vi "WriteFlattenImageOptions.vi"(8 "error in":errorcluster, 9 "Type of Flatten":T1 items=["Image", "Image and Vision Info", "Reference to Image"], 10 "Quality":i32=750, 11 "Compression (None)":T2 items=["None", "JPEG", "PACKED BINARY"]) -> (0 "error out":errorcluster)   [LabVIEW 2020, in "OpenLvVision_Image.lvlib" / "DataAccess.lvlib"]
doc: "These options dictate how images are compressed when converted to a string using the LabVIEW \"Flatten To String\" function."
uses:
  DataAccess.lvlib
  TypeDef/FlattenCompression.ctl
  TypeDef/TypeOfFlatten.ctl
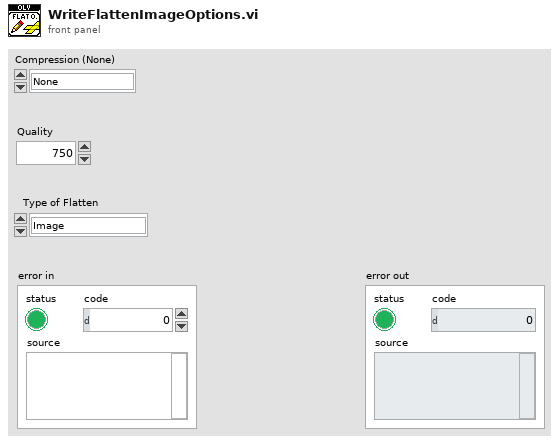
[diagram p1: front panel]
types:
  T1 = typedef "OpenLvVision_Image.lvlib/DataAccess.lvlib/TypeOfFlatten.ctl" = i32
  T2 = typedef "OpenLvVision_Image.lvlib/DataAccess.lvlib/FlattenCompression.ctl" = i32
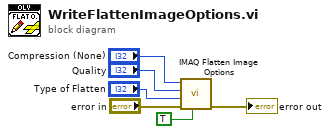
[diagram p0: block diagram]
diagram:
  n1 = call "IMAQ Flatten Image Options"("Get/Set Status? (Set)"=TRUE, "error in (no error)"="error in", "Type of Flatten (Image and Vision Info)"="Type of Flatten", "Quality (750)"="Quality", "Compression (None)"="Compression (None)") -> ("error out"=→"error out":errorcluster)  [unwired: 3 in, 3 out]
